vi "TimeSyncClient_Exec.vi"(8 "error in (no error)":errorcluster, 11 "ServerIPAddress":string="10.99.99.2") -> ()   [LabVIEW 2019, in "PhotonVisionLib.lvlib"]
doc: "Execute a PhotonVision Time Sync Client. Once a second it sends a UDP broadcast ping and listens for a response. If a good response is received, an FPGA time offset is calculated.\n\nThis VI contains a loop. Do not place this in another loop.\n\nThis routine is for diagnostic purposes. Robot code does NOT need this routine.\n\nInputs:\n -- Error In -- Optional error input cluster.\n\nOutputs:\n -- <None>"
uses:
  PhotonVisionLib.lvlib
  <vilib>/Rock Robotics/WPI/ThirdParty/JAS_Junk/TrajLib/VI/Util_GetTime_U32.vi
  PhotonVision_Globals.vi
  <vilib>/Rock Robotics/WPI/ThirdParty/JAS_Junk/TrajLib/VI/Util_GetTime_U64.vi
  <vilib>/Rock Robotics/WPI/ThirdParty/JAS_Junk/TrajLib/Trajectory_Library.lvlib
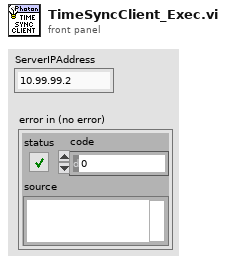
[diagram p1: front panel]
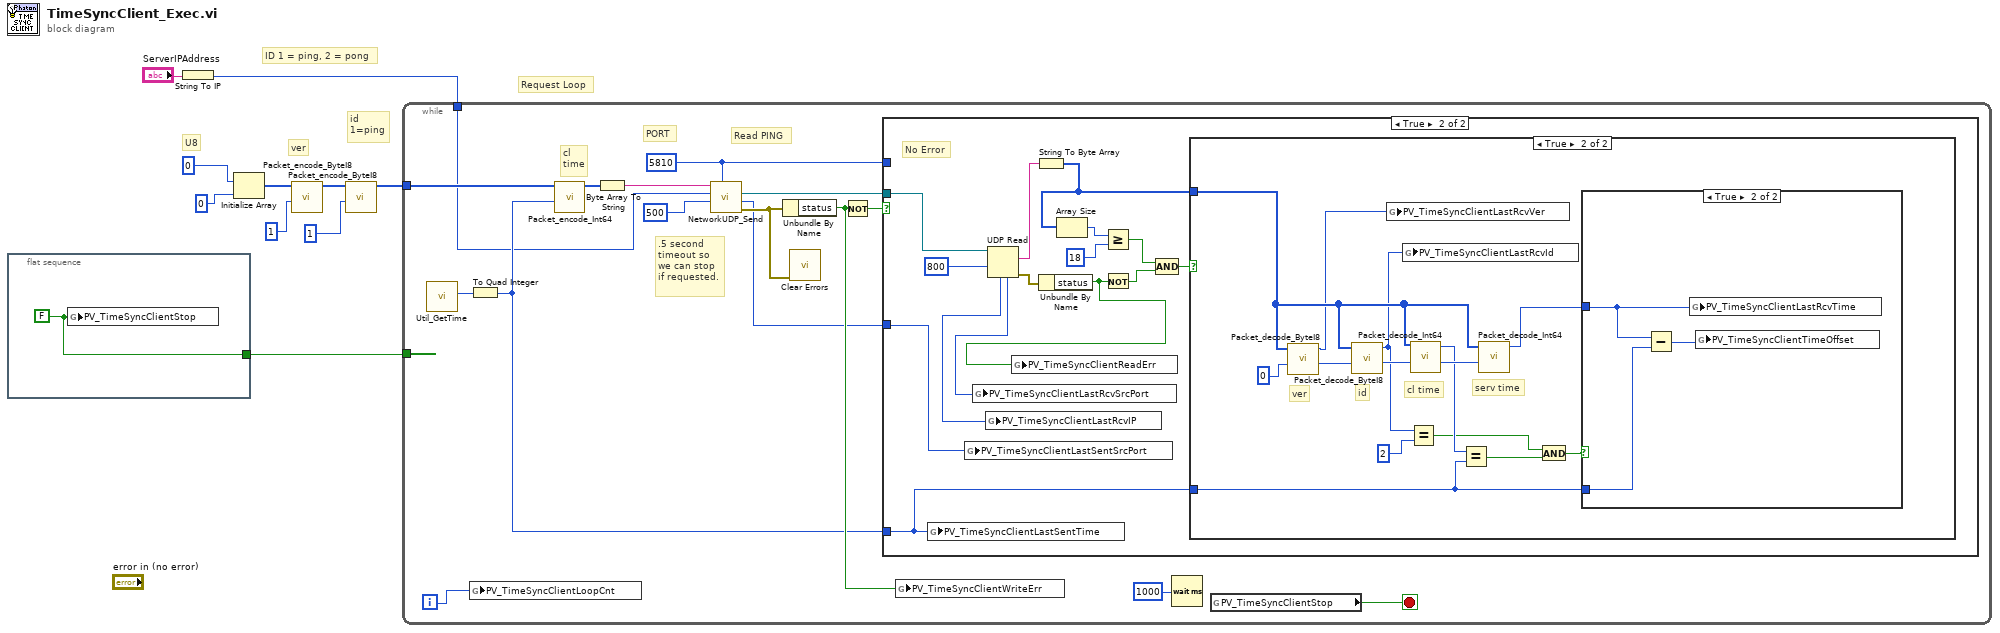
[diagram p0: block diagram]
diagram:
  # "Request Loop"
  # "ID 1 = ping, 2 = pong"
  # "id\n1=ping"
  # "ver"
  # "U8"
  n1 = flat-sequence {
    tunnel: [w11] -> w10
    frame #0 {
      w11 = FALSE ("PV_TimeSyncStopServ")
      n2 = global write "PhotonVision_Globals.vi" "PV_TimeSyncClientStop"(w11) -> ()
    }
  }
  n3 = String To IP(1:"ServerIPAddress") -> (0:w2:u32)
  n4 = Initialize Array(u8 0 ("element"), 0 ("dimension size")) -> (w9:u8[])
  n5 = call "Packet_encode_ByteI8.vi"("Int8_Value"=i8 1, "RawData In"=w9) -> ("RawData Out"=w8:u8[])  [unwired: 9 in]
  n6 = call "Packet_encode_ByteI8.vi"("Int8_Value"=i8 1, "RawData In"=w8) -> ("RawData Out"=w3:u8[])  [unwired: 9 in]
  n7 = while {
    tunnel: w10 -> [_]
    tunnel: w3 -> [w19]
    tunnel: w2 -> [w14]
    i -> [w25]
    stop <- w26 stop-if-true
    w12 = u16 5810 ("receiver port")
    # "cl\ntime"
    # "Read PING"
    # "PORT"
    # ".5 second\ntimeout so\nwe can stop\nif requested."
    n8 = call <vilib>:"Util_GetTime.vi"() -> ("FPGA_Time_MicroSeconds"=w18:u64)  [unwired: 9 in, 2 out]
    n9 = To Quad Integer(1:w18) -> (0:w16:i64)
    n10 = global write "PhotonVision_Globals.vi" "PV_TimeSyncClientLoopCnt"(w25) -> ()
    n11 = call "Packet_encode_Int64.vi"("Int64_Value"=w16, "RawData In"=w19) -> ("RawData Out"=w23:u8[])  [unwired: 9 in]
    n12 = Byte Array To String(unsigned byte array=w23) -> (string=w22:string)
    n13 = call <vilib>:"NetworkUDP_Send.vi"("remote port"=w12, "timeout ms (25000)"=500, "IP4 Address"=w14, "data string"=w22) -> ("error out"=w24:errorcluster, "LocalPort"=w13:u16, "UDP Network Connection out"=w15:refnum<k16>)  [unwired: 4 in, 1 out]
    n14 = Unbundle By Name(w24) -> ("status"=w21:bool)
    n15 = call <vilib>:"Clear Errors.vi"("error in (no error)"=w24) -> ()  [unwired: 5 in, 2 out]
    n16 = Not(x=w21) -> (.not. x?=w20:bool)
    n17 = case shown="True" w20 {
      tunnel: w16 -> [_ w31]
      tunnel: w15 -> [_ w42]
      tunnel: w13 -> [_ w28]
      tunnel: w12 -> [_ _]
      frame False {
      }
      frame True {
        # "No Error"
        n18 = global write "PhotonVision_Globals.vi" "PV_TimeSyncClientLastSentTime"(w31) -> ()
        n19 = global write "PhotonVision_Globals.vi" "PV_TimeSyncClientLastSentSrcPort"(w28) -> ()
        n20 = UDP Read(connection ID=w42, timeout ms (25000)=800) -> (data out=w37:string, error out=w40:errorcluster, 4:w30:u16, 6:w29:u32)  [unwired: 2 in, 1 out]
        n21 = global write "PhotonVision_Globals.vi" "PV_TimeSyncClientLastRcvSrcPort"(w30) -> ()
        n22 = global write "PhotonVision_Globals.vi" "PV_TimeSyncClientLastRcvIP"(w29) -> ()
        n23 = String To Byte Array(string=w37) -> (unsigned byte array=w33:u8[])
        n24 = Unbundle By Name(w40) -> ("status"=w32:bool)
        n25 = global write "PhotonVision_Globals.vi" "PV_TimeSyncClientReadErr"(w32) -> ()
        n26 = Array Size(array=w33) -> (size(s)=w39:i32)
        n27 = Greater Or Equal?(x=w39, y=18) -> (x >= y?=w36:bool)
        n28 = Not(x=w32) -> (.not. x?=w35:bool)
        n29 = Compound Arithmetic op=AND(w36, w35) -> (w34:bool)
        n30 = case shown="True" w34 {
          tunnel: w33 -> [_ w56]
          tunnel: w31 -> [_ w43]
          frame False {
          }
          frame True {
            # "serv time"
            # "cl time"
            # "id"
            # "ver"
            n31 = call "Packet_decode_ByteI8.vi"("StartByte"=0, "RawData"=w56) -> ("NextByte"=w54:i32, "Int8_Value"=w45:i8)  [unwired: 8 in]
            n32 = call "Packet_decode_ByteI8.vi"("StartByte"=w54, "RawData"=w56) -> ("NextByte"=w53:i32, "Int8_Value"=w44:i8)  [unwired: 8 in]
            n33 = global write "PhotonVision_Globals.vi" "PV_TimeSyncClientLastRcvVer"(w45) -> ()
            n34 = global write "PhotonVision_Globals.vi" "PV_TimeSyncClientLastRcvId"(w44) -> ()
            n35 = Equal?(x=w44, y=i8 2) -> (x = y?=w47:bool)
            n36 = call "Packet_decode_Int64.vi"("StartByte"=w53, "RawData"=w56) -> ("NextByte"=w51:i32, "Int64_Value"=w49:i64)  [unwired: 8 in]
            n37 = Equal?(x=w49, y=w43) -> (x = y?=w46:bool)
            n38 = call "Packet_decode_Int64.vi"("StartByte"=w51, "RawData"=w56) -> ("Int64_Value"=w52:i64)  [unwired: 8 in, 1 out]
            n39 = And(x=w47, y=w46) -> (x .and. y?=w48:bool)
            n40 = case shown="True" w48 {
              tunnel: w52 -> [_ w59]
              tunnel: w43 -> [_ w58]
              frame False {
              }
              frame True {
                n41 = Subtract(x=w59, y=w58) -> (x-y=w57:i64)
                n42 = global write "PhotonVision_Globals.vi" "PV_TimeSyncClientLastRcvTime"(w59) -> ()
                n43 = global write "PhotonVision_Globals.vi" "PV_TimeSyncClientTimeOffset"(w57) -> ()
              }
            }
          }
        }
      }
    }
    n44 = global write "PhotonVision_Globals.vi" "PV_TimeSyncClientWriteErr"(w21) -> ()
    n45 = Wait (ms)(milliseconds to wait=u32 1000) -> ()  [unwired: 1 out]
    n46 = global read "PhotonVision_Globals.vi" "PV_TimeSyncClientStop"() -> (w26:bool)
  }
